vi "Full Range Demo.vi"() -> ()   [LabVIEW 2012]
uses:
  LabVIEW/user.lib/SpectralRadar.llb/set Apodized Spectrum Output.vi
  LabVIEW/user.lib/SpectralRadar.llb/set Hor Mirrored Scan Output.vi
  LabVIEW/user.lib/SpectralRadar.llb/display Data 2D.vi
  LabVIEW/user.lib/SpectralRadar.llb/OCT Device.lvclass
  LabVIEW/user.lib/SpectralRadar.llb/Probe.lvclass
  LabVIEW/user.lib/SpectralRadar.llb/Processing.lvclass
  LabVIEW/user.lib/SpectralRadar.llb/Raw Data.lvclass
  LabVIEW/user.lib/SpectralRadar.llb/Data.lvclass
  LabVIEW/user.lib/SpectralRadar.llb/Scan Pattern.lvclass
  LabVIEW/user.lib/SpectralRadar.llb/FullRange.lvclass
  LabVIEW/user.lib/SpectralRadar.llb/Complex Data.lvclass
panel:
  in  "Cut Off":sgl
  out "Intensity Graph":dbl[][](graph)
  in  "stop":bool
  out "Spectral Data":dbl[][](graph)
  in  "AScans":i32=512
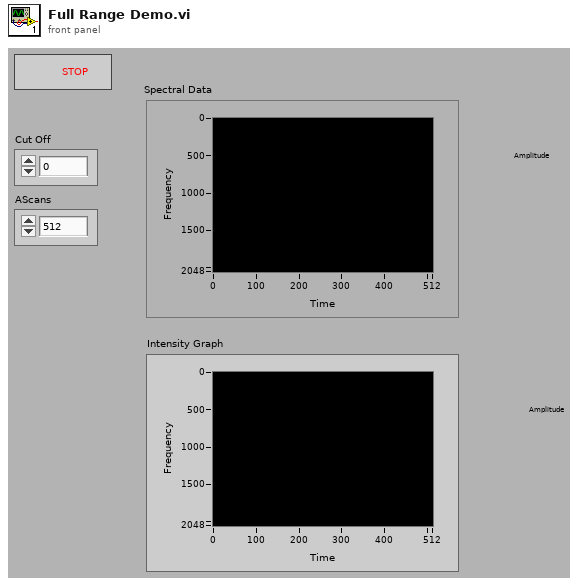
[diagram p1: front panel]
types:
  T1 = enum16{"Asynchronous Continuous", "Asynchronous Finite", "Synchronous"}
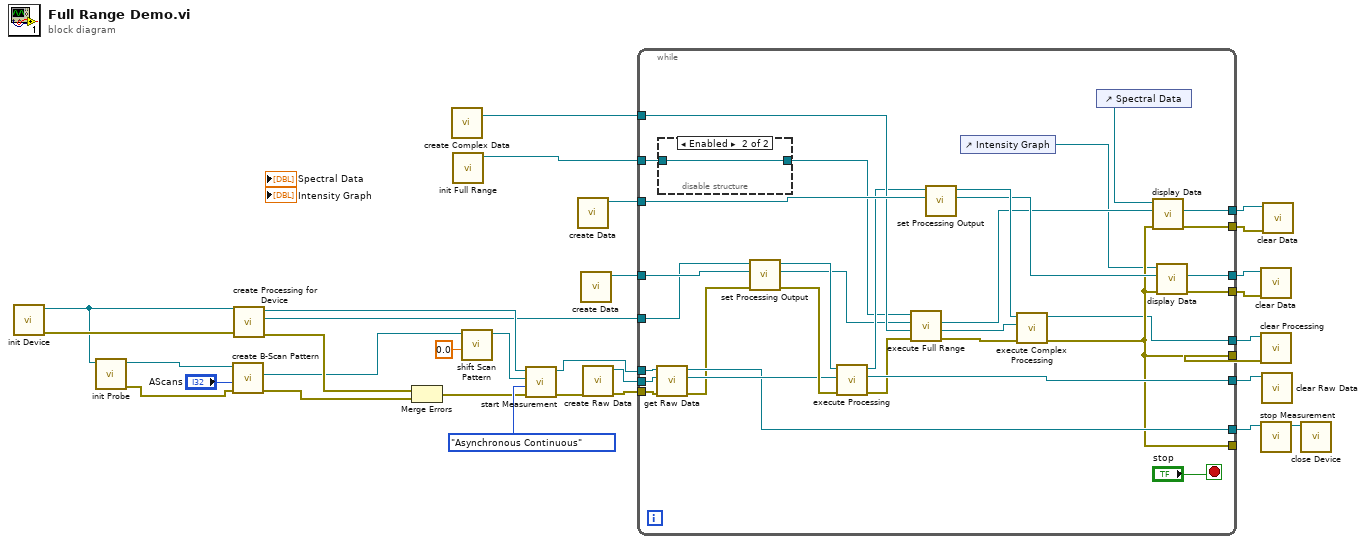
[diagram p0: block diagram]
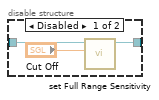
[diagram p2: hidden frame]
diagram:
  n1 = call "init Device.vi"() -> ("error out"=w31:errorcluster, "OCTDevice"=w16:refnum<class "OCT Device.lvclass">)  [unwired: 6 in]
  n2 = call "init Probe.vi"("OCT Device"=w16) -> ("error out"=w15:errorcluster, "GalvoControl"=w30:refnum<class "Probe.lvclass">)  [unwired: 5 in]
  n3 = call "create B-Scan Pattern.vi"("error in (no error)"=w15, "AScans"="AScans", "Probe"=w30) -> ("error out"=w27:errorcluster, "Scan Pattern"=w9:refnum<class "Scan Pattern.lvclass">)  [unwired: 3 in, 1 out]
  n4 = call "create Processing for Device.vi"("error in (no error)"=w31, "OCTDevice"=w16) -> ("error out"=w25:errorcluster, "Processing"=w20:refnum<class "Processing.lvclass">, "OCTDevice"=w21:refnum<class "OCT Device.lvclass">)  [unwired: 3 in]
  n5 = Merge Errors(w25, w27) -> (w26:errorcluster)
  n6 = call "create Complex Data.vi"() -> ("Complex Data"=w10:refnum<class "Complex Data.lvclass">)  [unwired: 2 in, 1 out]
  n7 = call "init Full Range.vi"() -> ("Full Range"=w11:refnum<class "FullRange.lvclass">)  [unwired: 6 in, 1 out]
  n8 = call "shift Scan Pattern.vi"("Shift Y"=0.0, "Scan Pattern in"=w9) -> ("Scan Pattern out"=w8:refnum<class "Scan Pattern.lvclass">)  [unwired: 4 in, 1 out]
  n9 = call "start Measurement.vi"("error in (no error)"=w26, "Acquisition Type"=T1."Asynchronous Continuous", "Scan Pattern"=w8, "OCTDevice"=w21) -> ("error out"=w23:errorcluster, "OCTDevice"=w12:refnum<class "OCT Device.lvclass">)  [unwired: 1 in, 1 out]
  n10 = call "create Data.vi"() -> ("Data"=w2:refnum<class "Data.lvclass">)  [unwired: 6 in, 1 out]
  n11 = call "create Data.vi"() -> ("Data"=w1:refnum<class "Data.lvclass">)  [unwired: 6 in, 1 out]
  n12 = call "create Raw Data.vi"("error in (no error)"=w23) -> ("error out"=w22:errorcluster, "Raw Data"=w24:refnum<class "Raw Data.lvclass">)  [unwired: 5 in]
  n13 = while {
    tunnel: w24 -> [w62]
    tunnel: w12 -> [w63]
    tunnel: w22 -> [w61]
    tunnel: w20 -> [w59]
    tunnel: w1 -> [w60]
    tunnel: [w55] -> w19
    tunnel: [w35] -> w18
    tunnel: [w54] -> w4
    tunnel: [w53] -> w6
    tunnel: [w52] -> w3
    tunnel: [w51] -> w5
    tunnel: [w50] -> w14
    tunnel: [w38] -> w17
    tunnel: [w38] -> _
    tunnel: w2 -> [w47]
    tunnel: w11 -> [w33]
    tunnel: w10 -> [w45]
    stop <- "stop" stop-if-true
    n14 = call "get Raw Data.vi"("error in (no error)"=w61, "RawData in"=w62, "OCTDevice in"=w63) -> ("error out"=w48:errorcluster, "RawData out"=w57:refnum<class "Raw Data.lvclass">, "OCTDevice out"=w50:refnum<class "OCT Device.lvclass">)  [unwired: 2 in]
    n15 = disable-structure shown="Enabled" {
      disable-tunnel: w33 -> [w66 w67]
      disable-tunnel: [w65 w67] -> w32
      frame Disabled {
        n16 = call "set Full Range Sensitivity.vi"("Cut Off"="Cut Off", "FullRange in"=w66) -> ("FullRange out"=w65:refnum<class "FullRange.lvclass">)  [unwired: 4 in, 1 out]
      }
      frame Enabled {
      }
    }
    n17 = call-poly "set Processing Output.vi"("error in (no error)"=w48, "Data"=w60, "Processing"=w59) -> ("error out"=w58:errorcluster, "Data"=w41:refnum<class "Data.lvclass">, "Processing"=w44:refnum<class "Processing.lvclass">)  [unwired: 2 in]
    n18 = call "execute Processing.vi"("error in (no error)"=w58, "Raw Data"=w57, "Processing"=w44) -> ("error out"=w46:errorcluster, "Raw Data"=w55:refnum<class "Raw Data.lvclass">, "Processing"=w43:refnum<class "Processing.lvclass">)  [unwired: 2 in]
    n19 = call "execute Full Range.vi"("error in (no error)"=w46, "Complex Data"=w45, "Data"=w41, "FullRange in"=w32) -> ("error out"=w39:errorcluster, "Complex Data 2"=w37:refnum<class "Complex Data.lvclass">, "Data 2"=w36:refnum<class "Data.lvclass">)  [unwired: 1 out]
    n20 = call-poly "set Processing Output.vi"("Data"=w47, "Processing"=w43) -> ("Data"=w40:refnum<class "Data.lvclass">, "Processing"=w42:refnum<class "Processing.lvclass">)  [unwired: 3 in, 1 out]
    n21 = control-ref of="Intensity Graph"() -> (w34:refnum<vi>)
    n22 = call "execute Complex Processing.vi"("error in (no error)"=w39, "Complex Data"=w37, "Processing"=w42) -> ("error out"=w38:errorcluster, "Processing"=w35:refnum<class "Processing.lvclass">)  [unwired: 2 in, 1 out]
    n23 = control-ref of="Spectral Data"() -> (w56:refnum<vi>)
    n24 = call-poly "display Data.vi"("error in (no error)"=w38, "Data in"=w36, "IntGraph Refnum"=w56) -> ("error out"=w51:errorcluster, "Data out"=w53:refnum<class "Data.lvclass">)  [unwired: 2 in, 1 out]
    n25 = call-poly "display Data.vi"("error in (no error)"=w38, "Data in"=w40, "IntGraph Refnum"=w34) -> ("error out"=w52:errorcluster, "Data out"=w54:refnum<class "Data.lvclass">)  [unwired: 2 in, 1 out]
  }
  n26 = call "clear Data.vi"("error in (no error)"=w3, "Data"=w4) -> ()  [unwired: 5 in, 1 out]
  n27 = call "clear Processing.vi"("error in (no error)"=w17, "Processing"=w18) -> ()  [unwired: 5 in, 1 out]
  n28 = call "stop Measurement.vi"("OCTDevice"=w14) -> ("OCTDevice"=w13:refnum<class "OCT Device.lvclass">)  [unwired: 5 in, 1 out]
  n29 = call "clear Raw Data.vi"("Raw Data"=w19) -> ()  [unwired: 6 in, 1 out]
  n30 = call "clear Data.vi"("error in (no error)"=w5, "Data"=w6) -> ()  [unwired: 5 in, 1 out]
  n31 = call "close Device.vi"("OCTDevice"=w13) -> ()  [unwired: 6 in, 1 out]
